vi "Leading Edge Detector.vi"(1 "Boolean":bool) -> (0 "Out":bool)   [LabVIEW 2019]
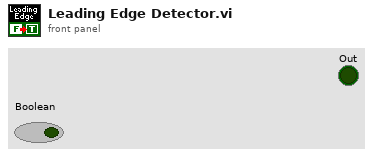
[diagram p1: front panel]
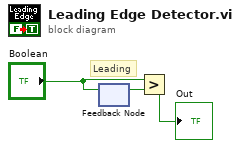
[diagram p0: block diagram]
diagram:
  # "Leading"
  n1 = feedback #1() -> (w3:bool)  [unwired: 1 in]
  n2 = feedback-in #1("Boolean") -> ()
  n3 = Greater?(x="Boolean", y=w3) -> (0:→"Out":bool)
